vi "GE 5565PIORC.Write VISA 5565.vi"(8 "error in (no error)":errorcluster, 10 "VISA 5565":refnum<visa-resource-name>, 11 "GE 5565PIORC in":refnum<class "GE 5565PIORC.lvclass">) -> (0 "error out":errorcluster, 3 "GE 5565PIORC out":refnum<class "GE 5565PIORC.lvclass">)   [LabVIEW 2017, in "GE 5565PIORC.lvclass"]
uses:
  GE 5565PIORC.lvclass
  GE 5565PIORC.lvclass/GE 5565PIORC.ctl
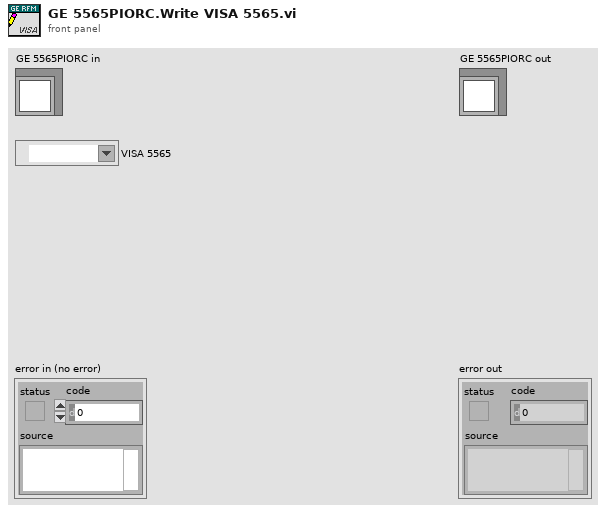
[diagram p1: front panel]
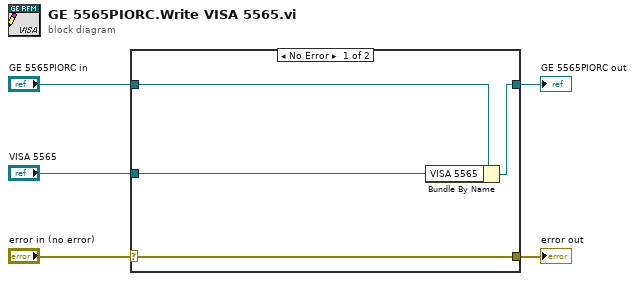
[diagram p0: block diagram]
diagram:
  n1 = case shown="No Error" "error in (no error)" {
    selector: "error in (no error)" -> [w9 w10]
    tunnel: [w9 w10] -> w4
    tunnel: [w7 w11] -> w2
    tunnel: "GE 5565PIORC in" -> [w8 w11]
    tunnel: "VISA 5565" -> [w6 _]
    frame No Error {
      n2 = Bundle By Name(cluster=w8, "VISA 5565"=w6) -> (w7:refnum<class "GE 5565PIORC.lvclass">)
    }
    frame Error {
    }
  }
  "error out" <- w4
  "GE 5565PIORC out" <- w2
